vi "Pre Launch Init.vi"(11 "Channel in":refnum<class "Channel.lvclass">) -> (0 "error out":errorcluster, 3 "Channel out":refnum<class "Channel.lvclass">)   [LabVIEW 2015, in "Channel.lvlib" / "Channel.lvclass"]
doc: "(<B>Filename</B>: Actor Framework.lvlib:Actor.lvclass:Pre Launch Init.vi)\n\nDefines behavior that occurs after the Launch Actor method is invoked but before the actor's Actor Core method begins running.\n\nThe Pre Launch Init method is guaranteed to finish before the Launch Actor method returns to its caller and before the actor itself receives any messages. Any references that the Pre Launch Init method obtains are guaranteed to have the same lifetime as the actor itself. Any errors that the Pre Launch Init method returns will abort the launch.\n\nBy default, this method does nothing. A descendant class may override it to define behavior."
uses:
  Channel.lvclass
  ChannelInfo.lvclass
  ChannelData.lvclass
  <userlib>/_Win8uiFramework/ViewableActor.lvclass
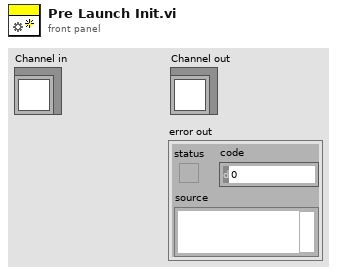
[diagram p1: front panel]
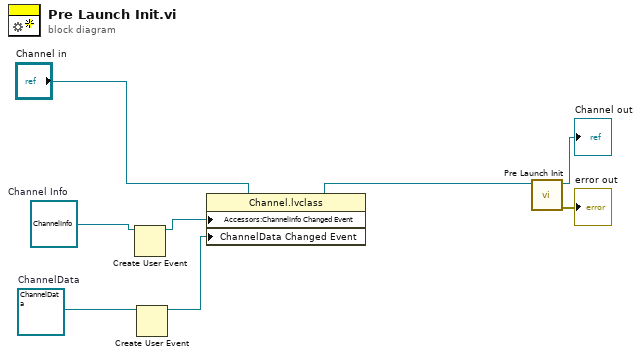
[diagram p0: block diagram]
diagram:
  w2 = refnum<class "ChannelData.lvclass"> refnum  # ChannelData
  w4 = refnum<class "ChannelInfo.lvclass"> refnum  # Channel Info
  n1 = Create User Event(user event datatype=w4) -> (user event=w3:refnum<user-event>)  [unwired: 1 in, 1 out]
  n2 = Create User Event(user event datatype=w2) -> (user event=w1:refnum<user-event>)  [unwired: 1 in, 1 out]
  n3 = property class="Channel.lvclass"(reference="Channel in", "Accessors:ChannelInfo Changed Event"=w3, "ChannelData Changed Event"=w1) -> (reference out=w5:refnum<class "Channel.lvclass">)  [unwired: 1 in, 1 out]
  n4 = call-parent "Pre Launch Init.vi"("ViewableActor in"=w5) -> ("error out"=→"error out":errorcluster, "ViewableActor out"=→"Channel out":refnum<class "Channel.lvclass">)  [unwired: 9 in]
